vi "CLUSTERBytePack.vi"() -> ()   [LabVIEW 2023]
doc: "This function takes a cluster that contains a DBL, Boolean, and I32 (in that order) as input. It squares the value of the DBL, halves the value of the I32, and inverts the Boolean. The result is returned in output.\n\nFor information on the data types used for the DLL function, right-click on the Call Library Function node and choose Configure."
uses:
  CLF_Example.dll
panel:
  out "output (8-byte spacing adjusted)":cluster{"DBL":dbl, "Boolean":bool, "I32":i32}={"DBL"=10.0, "Boolean"=FALSE, "I32"=5}
  out "output (8-byte spacing)":cluster{"DBL":dbl, "Boolean":bool, "I32":i32}={"DBL"=10.0, "Boolean"=FALSE, "I32"=5}
  out "output (1-byte spacing)":cluster{"DBL":dbl, "Boolean":bool, "I32":i32}={"DBL"=10.0, "Boolean"=FALSE, "I32"=5}
  in  "input":cluster{"DBL":dbl, "Boolean":bool, "I32":i32}={"DBL"=10.0, "Boolean"=FALSE, "I32"=5}
  # "See the block diagram for more information."
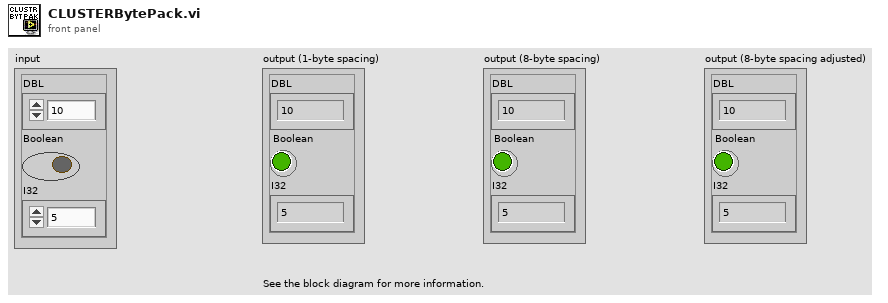
[diagram p1: front panel]
types:
  T1 = cluster{"DBL":dbl, "Boolean":bool, "I8":i8, "I16":i16, "I32":i32}
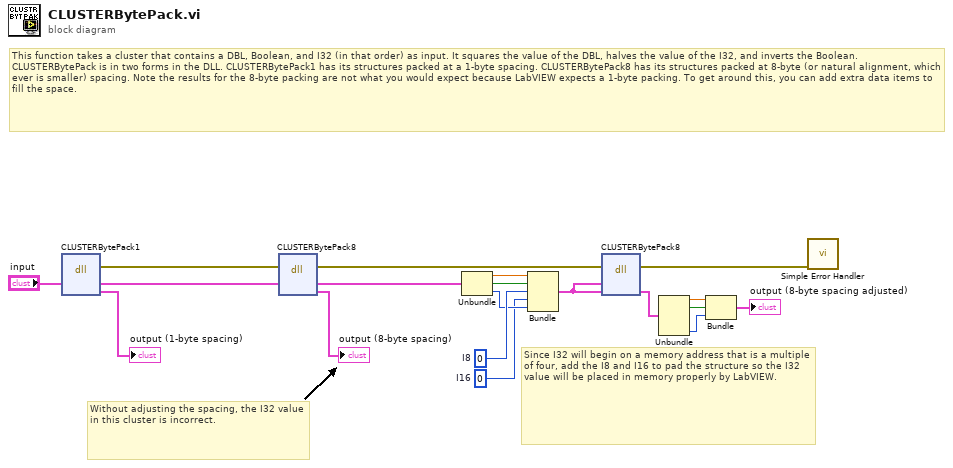
[diagram p0: block diagram]
diagram:
  w5 = i16 0  # I16
  w7 = i8 0  # I8
  # "Without adjusting the spacing, the I32 value in this cluster is incorrect."
  # "Since I32 will begin on a memory address that is a multiple of four, add the I8 and I16 to pad the structure so the I32 value will be placed in memory properly by LabVIEW."
  # "This function takes a cluster that contains a DBL, Boolean, and I32 (in that order) as input. It squares the value of the DBL, halves the value of the I32, and inverts the Boolean. CLUSTERBytePack is in two forms in the DLL. CLUSTERBytePack1 has its structures packed at a 1-byte spacing. CLUSTERBytePack8 has its structures packed at 8-byte (or natural alignment, which ever is smaller) spacing. Note the results for the 8-byte packing are not what you would expect because LabVIEW expects a 1-byte packing. To get around this, you can add extra data items to fill the space."
  n1 = dll-call lib="c:/dev/_r/4/eng/lv-core/lvpostprocessingd/lv_mc_x86_64/dist_i386/examples/Connectivity/Libraries and Executables/DLL Calling VIs/CLF_Example**.*" fn="CLUSTERBytePack1"("input"="input") -> (error out=w3:errorcluster, "input"=w17:cluster{"DBL":dbl, "Boolean":bool, "I32":i32}, "output (1-byte spacing)"=→"output (1-byte spacing)":cluster{"DBL":dbl, "Boolean":bool, "I32":i32})  [unwired: 3 in, 3 out]
  n2 = dll-call lib="c:/dev/_r/4/eng/lv-core/lvpostprocessingd/lv_mc_x86_64/dist_i386/examples/Connectivity/Libraries and Executables/DLL Calling VIs/CLF_Example**.*" fn="CLUSTERBytePack8"(error in=w3, "input"=w17) -> (error out=w2:errorcluster, "input"=w15:cluster{"DBL":dbl, "Boolean":bool, "I32":i32}, "output (8-byte spacing)"=→"output (8-byte spacing)":cluster{"DBL":dbl, "Boolean":bool, "I32":i32})  [unwired: 2 in, 3 out]
  n3 = Unbundle(w15) -> ("DBL"=w14:dbl, "Boolean"=w13:bool, "I32"=w6:i32)
  n4 = Bundle("DBL"=w14, "Boolean"=w13, "I8"=w7, "I16"=w5, "I32"=w6) -> (w11:T1)  [unwired: 1 out]
  n5 = dll-call lib="c:/dev/_r/4/eng/lv-core/lvpostprocessingd/lv_mc_x86_64/dist_i386/examples/Connectivity/Libraries and Executables/DLL Calling VIs/CLF_Example**.*" fn="CLUSTERBytePack8"(error in=w2, "input"=w11, "output"=w11) -> (error out=w1:errorcluster, "output"=w12:T1)  [unwired: 2 in, 3 out]
  n6 = Unbundle(w12) -> ("DBL"=w10:dbl, "Boolean"=w9:bool, "I32"=w4:i32)  [unwired: 2 out]
  n7 = Bundle("DBL"=w10, "Boolean"=w9, "I32"=w4) -> (→"output (8-byte spacing adjusted)":cluster{"DBL":dbl, "Boolean":bool, "I32":i32})  [unwired: 1 out]
  n8 = call <vilib>:"Simple Error Handler.vi"("error in (no error)"=w1) -> ()  [unwired: 4 in, 5 out]
